vi "GT Buf Move.vi"(0 "cardNum":i16, 1 "vel":dbl, 2 "modal":i16, 5 "crd":i16, 7 "moveAxis":i16, 9 "pos":i32, 11 "error in (no error)":errorcluster caption="错误输入（无错误）", 12 "acc":dbl, 13 "fifo":i16) -> (4 "function return":i16, 15 "error out":errorcluster caption="错误输出")   [LabVIEW 2020, in "gts.lvlib"]
doc: "GT_API GT_BufMove(short cardNum,short crd,short moveAxis,long pos,double vel,double acc,short modal,short fifo=0);"
uses:
  gts.lvlib
  dll/32bit/multi_card/gts.dll
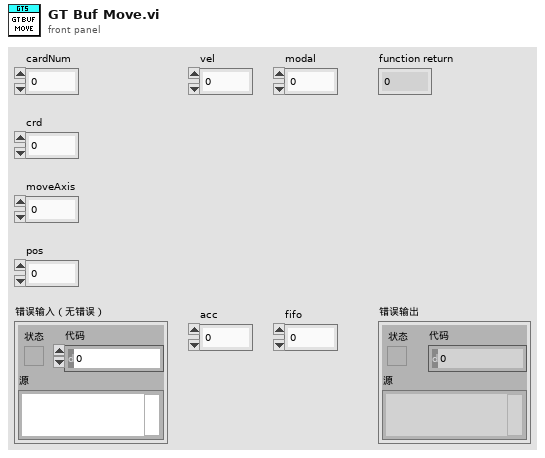
[diagram p1: front panel]
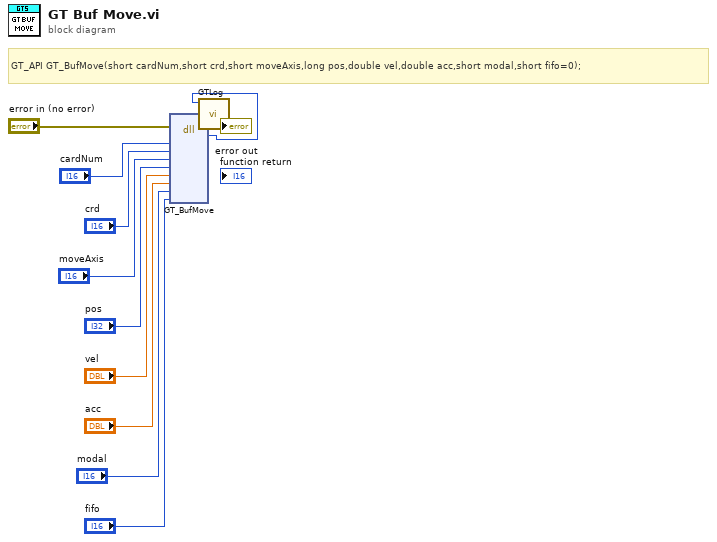
[diagram p0: block diagram]
diagram:
  # "GT_API GT_BufMove(short cardNum,short crd,short moveAxis,long pos,double vel,double acc,short modal,short fifo=0);"
  n1 = dll-call lib="C:/1228/dll/32bit/multi_card/gts.dll" fn="GT_BufMove"(error in="error in (no error)", "cardNum"="cardNum", "crd"="crd", "moveAxis"="moveAxis", "pos"="pos", "vel"="vel", "acc"="acc", "modal"="modal", "fifo"="fifo") -> (error out=w3:errorcluster, w1:i16)  [unwired: 10 in, 1 out]
  n2 = call "GTLog.vi"("error in (no error)"=w3, "Numeric"=w1) -> ("error out"=→"error out":errorcluster)  [unwired: 9 in]
